vi "FTW-Test-String-Random.vi"() -> (0 "Test Result":errorcluster)   [LabVIEW 2015]
panel:
  out "Array":string[](array[string])
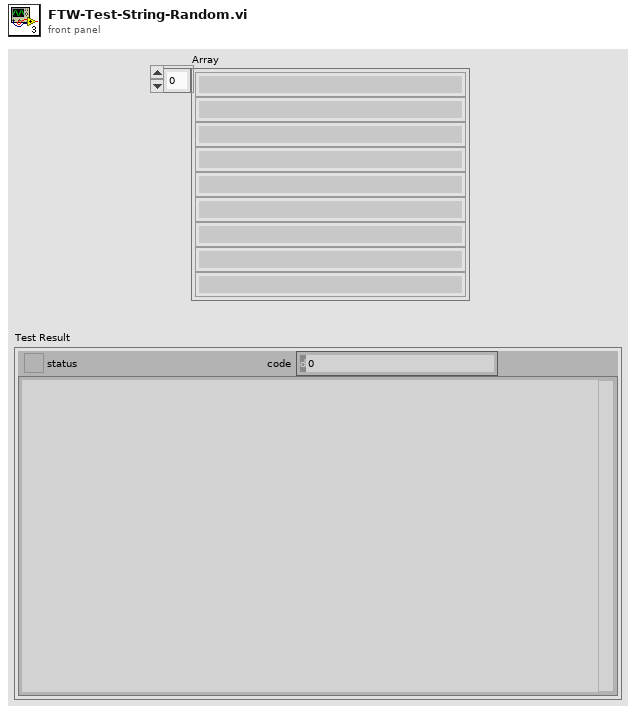
[diagram p1: front panel]
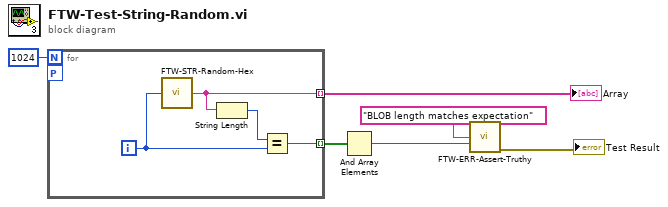
[diagram p0: block diagram]
diagram:
  n1 = for {
    N: 1024 -> [_]
    tunnel: [w7] -> w6 mode=indexing
    workers-P: _ -> [_]
    tunnel: [w9] -> w3 mode=indexing
    i -> [w8]
    n2 = call "FTW-STR-Random-Hex.vi"("String Length"=w8) -> ("Random Hex String"=w7:string)  [unwired: 3 in]
    n3 = String Length(string=w7) -> (length=w10:i32)
    n4 = Equal?(x=w10, y=w8) -> (x = y?=w9:bool)
  }
  "Array" <- w6
  n5 = And Array Elements(Boolean array=w3) -> (logical AND=w2:bool)
  n6 = call "FTW-ERR-Assert-Truthy.vi"("Assertion"="BLOB length matches expectation", "Assertion holds true?"=w2) -> ("error out"=→"Test Result":errorcluster)  [unwired: 13 in]
